vi "Vi_MotorisationManuelle.vi"(0 "x+":bool, 1 "Vitesse Manuelle Y":dbl, 2 "Vitesse Manuelle X":dbl, 3 "x-":bool, 5 "?":bool, 7 "x+y+":bool, 9 "x-y+":bool, 10 "Remise a zero X":bool, 12 "x+y-":bool, 13 "y+":bool, 14 "?":bool, 15 "Remise a zero Y":bool) -> (4 "Connecté":bool, 6 "Deverouillé":bool)   [LabVIEW 2015]
uses:
  Variable globale.vi
  <userlib>/ICNC/ICNC2.lvlib
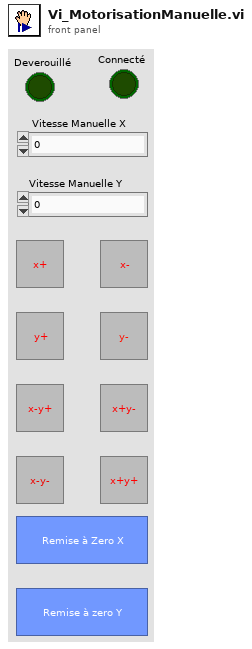
[diagram p1: front panel]
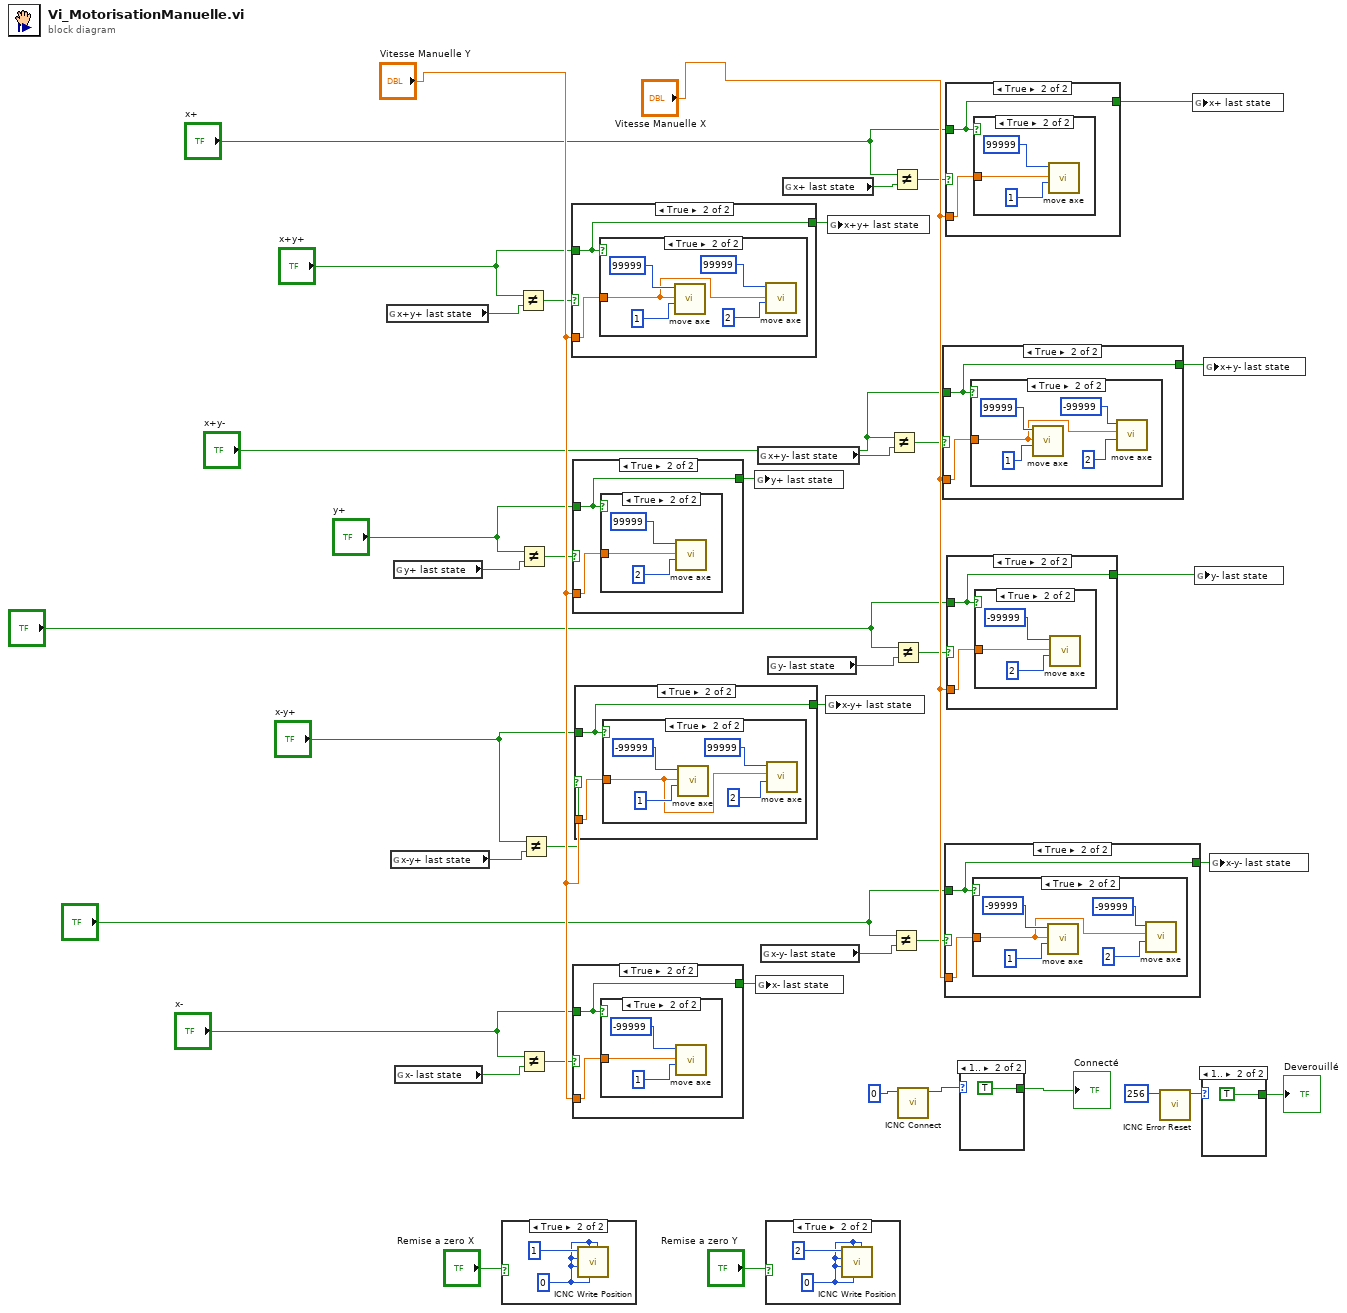
[diagram p0: block diagram]
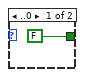
[diagram p2: hidden frame]
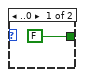
[diagram p3: hidden frame]
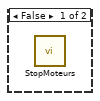
[diagram p7: hidden frame]
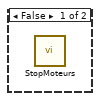
[diagram p9: hidden frame]
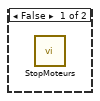
[diagram p11: hidden frame]
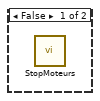
[diagram p13: hidden frame]
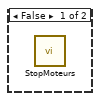
[diagram p15: hidden frame]
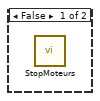
[diagram p17: hidden frame]
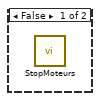
[diagram p19: hidden frame]
diagram:
  n1 = global read "Variable globale.vi" "x+y+ last state"() -> (w14:bool)
  n2 = global read "Variable globale.vi" "x-y+ last state"() -> (w30:bool)
  n3 = global read "Variable globale.vi" "y+ last state"() -> (w22:bool)
  n4 = global read "Variable globale.vi" "x- last state"() -> (w18:bool)
  n5 = case shown="True" "Remise a zero X" {
    frame False {
    }
    frame True {
      w43 = 0
      n6 = call <userlib>:"ICNC Write Position.vi"("PositionB"=w43, "PositionA"=w43, "PositionZ"=w43, "PositionY"=w43, "PositionX"=w43, "Axis"=1) -> ()  [unwired: 4 in, 2 out]
    }
  }
  n7 = Not Equal?(x="x+y+", y=w14) -> (x != y?=w13:bool)
  n8 = Not Equal?(x="y+", y=w22) -> (x != y?=w21:bool)
  n9 = Not Equal?(x="x-", y=w18) -> (x != y?=w17:bool)
  n10 = Not Equal?(x="x-y+", y=w30) -> (x != y?=w29:bool)
  n11 = case shown="True" w13 {
    tunnel: "Vitesse Manuelle Y" -> [_ w47]
    tunnel: "x+y+" -> [w45 w46]
    tunnel: [w45 w46] -> w15
    frame False {
    }
    frame True {
      n12 = case shown="True" w46 {
        tunnel: w47 -> [_ w49]
        frame False {
          n13 = call "StopMoteurs.vi"() -> ()  [unwired: 12 in]
        }
        frame True {
          n14 = call "move axe.vi"("Axe"=1, "Vitesse"=w49, "Angle"=99999) -> ()  [unwired: 9 in]
          n15 = call "move axe.vi"("Axe"=2, "Vitesse"=w49, "Angle"=99999) -> ()  [unwired: 9 in]
        }
      }
    }
  }
  n16 = case shown="True" w21 {
    tunnel: "Vitesse Manuelle Y" -> [_ w55]
    tunnel: "y+" -> [w53 w54]
    tunnel: [w53 w54] -> w23
    frame False {
    }
    frame True {
      n17 = case shown="True" w54 {
        tunnel: w55 -> [_ w57]
        frame False {
          n18 = call "StopMoteurs.vi"() -> ()  [unwired: 12 in]
        }
        frame True {
          n19 = call "move axe.vi"("Axe"=2, "Vitesse"=w57, "Angle"=99999) -> ()  [unwired: 9 in]
        }
      }
    }
  }
  n20 = case shown="True" w17 {
    tunnel: "Vitesse Manuelle Y" -> [_ w61]
    tunnel: "x-" -> [w59 w60]
    tunnel: [w59 w60] -> w19
    frame False {
    }
    frame True {
      n21 = case shown="True" w60 {
        tunnel: w61 -> [_ w63]
        frame False {
          n22 = call "StopMoteurs.vi"() -> ()  [unwired: 12 in]
        }
        frame True {
          n23 = call "move axe.vi"("Axe"=1, "Vitesse"=w63, "Angle"=-99999) -> ()  [unwired: 9 in]
        }
      }
    }
  }
  n24 = case shown="True" w29 {
    tunnel: "Vitesse Manuelle Y" -> [_ w67]
    tunnel: "x-y+" -> [w65 w66]
    tunnel: [w65 w66] -> w31
    frame False {
    }
    frame True {
      n25 = case shown="True" w66 {
        tunnel: w67 -> [_ w68]
        frame False {
          n26 = call "StopMoteurs.vi"() -> ()  [unwired: 12 in]
        }
        frame True {
          n27 = call "move axe.vi"("Axe"=1, "Vitesse"=w68, "Angle"=-99999) -> ()  [unwired: 9 in]
          n28 = call "move axe.vi"("Axe"=2, "Vitesse"=w68, "Angle"=99999) -> ()  [unwired: 9 in]
        }
      }
    }
  }
  n29 = global write "Variable globale.vi" "y+ last state"(w23) -> ()
  n30 = global write "Variable globale.vi" "x- last state"(w19) -> ()
  n31 = global read "Variable globale.vi" "x+y- last state"() -> (w26:bool)
  n32 = global read "Variable globale.vi" "x-y- last state"() -> (w38:bool)
  n33 = case shown="True" "Remise a zero Y" {
    frame False {
    }
    frame True {
      w73 = 0
      n34 = call <userlib>:"ICNC Write Position.vi"("PositionB"=w73, "PositionA"=w73, "PositionZ"=w73, "PositionY"=w73, "PositionX"=w73, "Axis"=2) -> ()  [unwired: 4 in, 2 out]
    }
  }
  n35 = global read "Variable globale.vi" "y- last state"() -> (w34:bool)
  n36 = global read "Variable globale.vi" "x+ last state"() -> (w10:bool)
  n37 = global write "Variable globale.vi" "x-y+ last state"(w31) -> ()
  n38 = global write "Variable globale.vi" "x+y+ last state"(w15) -> ()
  n39 = Not Equal?(x="x+y-", y=w26) -> (x != y?=w25:bool)
  n40 = Not Equal?(x="?", y=w38) -> (x != y?=w37:bool)
  n41 = Not Equal?(x="x+", y=w10) -> (x != y?=w9:bool)
  n42 = Not Equal?(x="?", y=w34) -> (x != y?=w33:bool)
  n43 = call <userlib>:"ICNC Connect.vi"("ICNC_Number"=0) -> ("function return"=w4:u32)  [unwired: 9 in, 1 out]
  n44 = case shown="True" w25 {
    tunnel: "Vitesse Manuelle X" -> [_ w77]
    tunnel: "x+y-" -> [w75 w76]
    tunnel: [w75 w76] -> w27
    frame False {
    }
    frame True {
      n45 = case shown="True" w76 {
        tunnel: w77 -> [_ w78]
        frame False {
          n46 = call "StopMoteurs.vi"() -> ()  [unwired: 12 in]
        }
        frame True {
          n47 = call "move axe.vi"("Axe"=1, "Vitesse"=w78, "Angle"=99999) -> ()  [unwired: 9 in]
          n48 = call "move axe.vi"("Axe"=2, "Vitesse"=w78, "Angle"=-99999) -> ()  [unwired: 9 in]
        }
      }
    }
  }
  n49 = case shown="True" w37 {
    tunnel: "Vitesse Manuelle X" -> [_ w85]
    tunnel: "?" -> [w83 w84]
    tunnel: [w83 w84] -> w39
    frame False {
    }
    frame True {
      n50 = case shown="True" w84 {
        tunnel: w85 -> [_ w86]
        frame False {
          n51 = call "StopMoteurs.vi"() -> ()  [unwired: 12 in]
        }
        frame True {
          n52 = call "move axe.vi"("Axe"=1, "Vitesse"=w86, "Angle"=-99999) -> ()  [unwired: 9 in]
          n53 = call "move axe.vi"("Axe"=2, "Vitesse"=w86, "Angle"=-99999) -> ()  [unwired: 9 in]
        }
      }
    }
  }
  n54 = case shown="True" w9 {
    tunnel: "Vitesse Manuelle X" -> [_ w93]
    tunnel: "x+" -> [w91 w92]
    tunnel: [w91 w92] -> w11
    frame False {
    }
    frame True {
      n55 = case shown="True" w92 {
        tunnel: w93 -> [_ w95]
        frame False {
          n56 = call "StopMoteurs.vi"() -> ()  [unwired: 12 in]
        }
        frame True {
          n57 = call "move axe.vi"("Axe"=1, "Vitesse"=w95, "Angle"=99999) -> ()  [unwired: 9 in]
        }
      }
    }
  }
  n58 = case shown="True" w33 {
    tunnel: "Vitesse Manuelle X" -> [_ w99]
    tunnel: "?" -> [w97 w98]
    tunnel: [w97 w98] -> w35
    frame False {
    }
    frame True {
      n59 = case shown="True" w98 {
        tunnel: w99 -> [_ w101]
        frame False {
          n60 = call "StopMoteurs.vi"() -> ()  [unwired: 12 in]
        }
        frame True {
          n61 = call "move axe.vi"("Axe"=2, "Vitesse"=w101, "Angle"=-99999) -> ()  [unwired: 9 in]
        }
      }
    }
  }
  n62 = case shown="1.." w4 {
    tunnel: [FALSE TRUE] -> w1
    frame ..0 {
    }
    frame 1.. {
    }
  }
  "Connecté" <- w1
  n63 = call <userlib>:"ICNC Error Reset.vi"("ErrorBits"=256) -> ("function return"=w5:u32)  [unwired: 9 in, 1 out]
  n64 = global write "Variable globale.vi" "x+ last state"(w11) -> ()
  n65 = global write "Variable globale.vi" "y- last state"(w35) -> ()
  n66 = case shown="1.." w5 {
    tunnel: [FALSE TRUE] -> w2
    frame ..0 {
    }
    frame 1.. {
    }
  }
  "Deverouillé" <- w2
  n67 = global write "Variable globale.vi" "x+y- last state"(w27) -> ()
  n68 = global write "Variable globale.vi" "x-y- last state"(w39) -> ()
